vi "Clock.vi"() -> ()   [LabVIEW 2014]
panel:
  out "Second":dbl
  out "Minute":dbl
  out "Hour":dbl
  in  "stop":bool
  out "XY Graph":cluster{dbl[], dbl[]}[](graph)
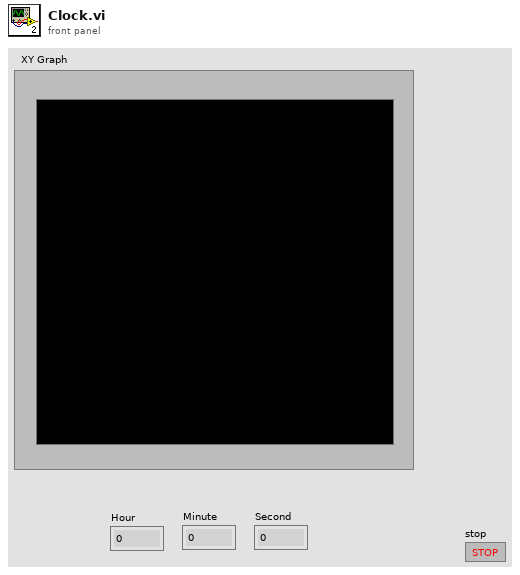
[diagram p1: front panel]
types:
  T1 = typedef "LVDateTimeRec.ctl" = cluster{"fractional second":dbl, "second":i32, "minute":i32, "hour":i32, "day of month":i32, "month":i32, "year":i32, "day of week":i32, "day of year":i32, "DST":i32}
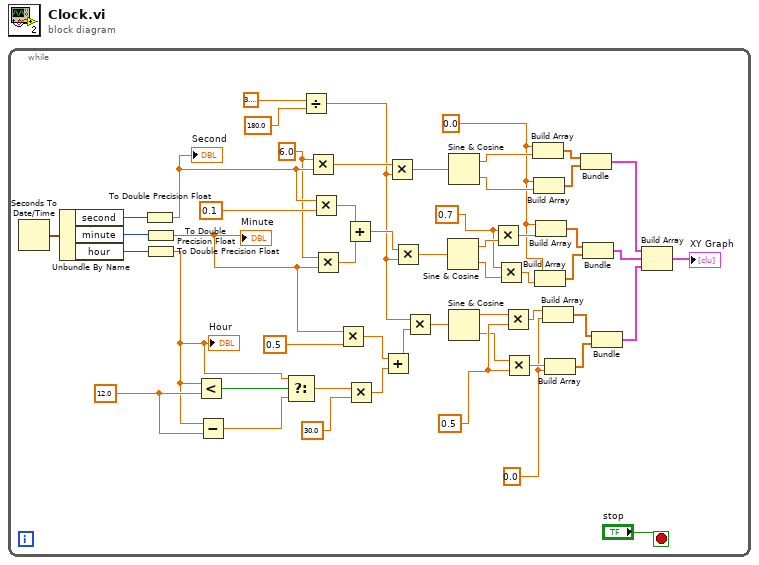
[diagram p0: block diagram]
diagram:
  n1 = while {
    stop <- "stop" stop-if-true
    w8 = 0.0
    w12 = 0.5
    w23 = 12.0
    w31 = 0.7
    w28 = 0.0
    w38 = 6.0
    n2 = Seconds To Date/Time() -> (date time rec=w52:T1)  [unwired: 2 in]
    n3 = Unbundle By Name(w52) -> ("second"=w51:i32, "minute"=w50:i32, "hour"=w49:i32)
    n4 = To Double Precision Float(number=w51) -> (double precision float=w40:dbl)
    "Second" <- w40
    n5 = To Double Precision Float(number=w50) -> (double precision float=w21:dbl)
    "Minute" <- w21
    n6 = To Double Precision Float(number=w49) -> (double precision float=w22:dbl)
    "Hour" <- w22
    n7 = Less?(x=w22, y=w23) -> (x < y?=w25:bool)
    n8 = Subtract(x=w22, y=w23) -> (x-y=w24:dbl)
    n9 = Select(t=w22, s=w25, f=w24) -> (s? t:f=w19:dbl)
    n10 = Divide(x=3.141592653589793, y=180.0) -> (x/y=w14:dbl)
    n11 = Multiply(x=w38, y=w40) -> (x*y=w46:dbl)
    n12 = Multiply(x=w40, y=0.1) -> (x*y=w36:dbl)
    n13 = Multiply(x=w38, y=w21) -> (x*y=w37:dbl)
    n14 = Multiply(x=w21, y=0.5) -> (x*y=w16:dbl)
    n15 = Add(x=w36, y=w37) -> (x+y=w35:dbl)
    n16 = Multiply(x=w19, y=30.0) -> (x*y=w17:dbl)
    n17 = Add(x=w16, y=w17) -> (x+y=w15:dbl)
    n18 = Multiply(x=w46, y=w14) -> (x*y=w45:dbl)
    n19 = Multiply(x=w35, y=w14) -> (x*y=w34:dbl)
    n20 = Multiply(x=w14, y=w15) -> (x*y=w13:dbl)
    n21 = Sine & Cosine(0:w34) -> (1:w33:dbl, 2:w32:dbl)
    n22 = Sine & Cosine(0:w45) -> (1:w44:dbl, 2:w42:dbl)
    n23 = Sine & Cosine(0:w13) -> (1:w10:dbl, 2:w11:dbl)
    n24 = Multiply(x=w31, y=w33) -> (x*y=w30:dbl)
    n25 = Multiply(x=w31, y=w32) -> (x*y=w29:dbl)
    n26 = Multiply(x=w10, y=w12) -> (x*y=w7:dbl)
    n27 = Multiply(x=w11, y=w12) -> (x*y=w9:dbl)
    n28 = Build Array(w28, w44) -> (w43:dbl[])
    n29 = Build Array(w28, w42) -> (w41:dbl[])
    n30 = Build Array(w28, w29) -> (w26:dbl[])
    n31 = Build Array(w28, w30) -> (w27:dbl[])
    n32 = Build Array(w7, w8) -> (w6:dbl[])
    n33 = Build Array(w9, w8) -> (w5:dbl[])
    n34 = Bundle(w43, w41) -> (w2:cluster{dbl[], dbl[]})  [unwired: 1 in]
    n35 = Bundle(w27, w26) -> (w3:cluster{dbl[], dbl[]})  [unwired: 1 in]
    n36 = Bundle(w6, w5) -> (w4:cluster{dbl[], dbl[]})  [unwired: 1 in]
    n37 = Build Array(w2, w3, w4) -> (→"XY Graph":cluster{dbl[], dbl[]}[])
  }
